vi "Divisor_String(SubVI).vi"(1 "read buffer":string) -> (0 "Cluster":T1)   [LabVIEW 2016]
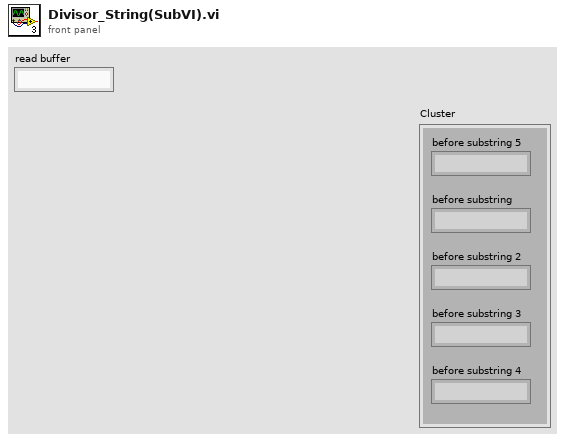
[diagram p1: front panel]
types:
  T1 = cluster{"before substring":string, "before substring 2":string, "before substring 3":string, "before substring 4":string, "before substring 5":string}
  T2 = cluster{"read buffer":string, "read buffer":string, "read buffer":string, "read buffer":string, "read buffer":string}
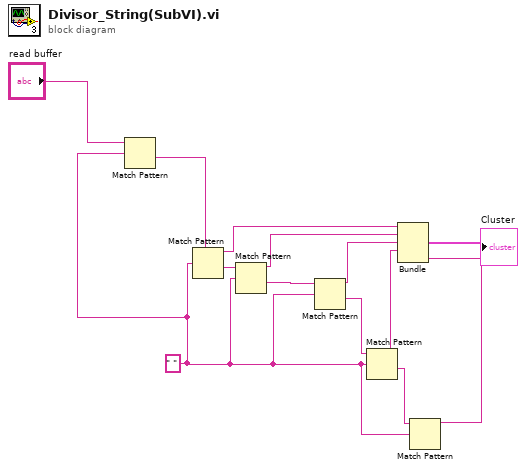
[diagram p0: block diagram]
diagram:
  w3 = " " ("regular expression")
  n1 = Match Pattern(string="read buffer", regular expression=w3) -> (after substring=w1:string)  [unwired: 1 in, 3 out]
  n2 = Match Pattern(string=w1, regular expression=w3) -> (before substring=w2:string, after substring=w10:string)  [unwired: 1 in, 2 out]
  n3 = Match Pattern(string=w10, regular expression=w3) -> (before substring=w8:string, after substring=w13:string)  [unwired: 1 in, 2 out]
  n4 = Match Pattern(string=w13, regular expression=w3) -> (before substring=w7:string, after substring=w12:string)  [unwired: 1 in, 2 out]
  n5 = Match Pattern(string=w12, regular expression=w3) -> (before substring=w6:string, after substring=w11:string)  [unwired: 1 in, 2 out]
  n6 = Match Pattern(string=w11, regular expression=w3) -> (before substring=w5:string)  [unwired: 1 in, 3 out]
  n7 = Bundle("read buffer"=w2, "read buffer"=w8, "read buffer"=w7, "read buffer"=w6, "read buffer"=w5) -> (→"Cluster":T2)  [unwired: 1 in]
